vi "PID_controller_21.vi"() -> ()   [LabVIEW 2011]
uses:
  <vilib>/Analysis/NI_AALPro.lvlib
panel:
  in  "|angle backlash|":dbl
  out "prev dAngle":dbl
  out "dAngle":dbl
  out "XY Graph 2":cluster{"Value":dbl[], "Value":dbl[]}(graph)
  out "Angle array":dbl[](array[numeric])
  in  "Move to ref angle first":bool=TRUE
  in  "time to wait (s)":dbl=2.0
  in  "angle backlash (deg)":dbl=5.0 format="%.1f"
  out "Polynomial Coefficients":dbl[](array[numeric])=[-1.4185856873488687, 0.3207828308209371, 0.13144453708617976]
  out "Best Polynomial Fit":dbl[](array[numeric])=[-1.4185856873488687, -1.6139263817489564, -1.4535753275096295, -0.934721257482187, -0.06084472416107456, 1.168009538292087, 2.7539547788012695, 4.6979090060566655, 6.9965349595828625, 9.65378216839643, 12.656869913925354, 16.032582856357365, 19.766321537116767, 23.839791139200322, 28.29201256813708, 33.090057519195085, 38.231169600301214, 43.741895001434145, 49.604230522561835, 55.817258155180305, 63.621549699110574, 70.69684374251437, 78.07805746158404, 85.78401348130417, 93.89514333055536, 102.37353612475415, 111.1585051750553, 120.33168859799997, 129.86351160527155, 139.71949074374146, 149.9584374415381, 160.56464392932688, 171.50086747103902, 182.82343196442633, 194.50463604214053, 206.47125485701025, 218.94296295023602, 231.70008578092185, 244.74755627283324, 258.3136303817438]
  out "tFit_array":dbl[](array[numeric])=[-2.0, 0.0]
  out "PFit_array":dbl[](array[numeric])=[73.96843433835814, 74.61000000000001]
  out "error array":dbl[](array[numeric])=[-1.3899999999999864, -1.7800000000000011, -1.3500000000000085, -0.6200000000000045, 0.5699999999999932, 1.6099999999999994, 1.1999999999999886, 0.3199999999999932, -0.13000000000000966, -1.3700000000000045, -1.9499999999999886, -1.7399999999999949, -1.1200000000000045, -0.11999999999999034, 1.759999999999991, 2.3500000000000085, 2.1700000000000017, 1.4099999999999966, 0.4299999999999926, -0.6500000000000057, 54.959999999999994, 55.099999999999994, 55.66000000000001, 56.55000000000001, 57.02000000000001, 58.03, 58.129999999999995, 57.11999999999999, 56.599999999999994, 55.47, 54.80000000000001, 54.84, 55.129999999999995, 55.58, 57.16000000000001, 58.11, 58.09, 57.510000000000005, 56.74000000000001, 55.709999999999994]
  out "dt array":dbl[](array[numeric])=[0.0, -1.1669999999867287, -2.3260000000009313, -3.4940000000060536, -4.657999999995809, -5.820999999996275, -6.98499999998603, -8.14999999999418, -9.314000000013039, -10.478999999992084, -11.64000000001397, -12.807000000000698, -13.973999999987427, -15.135999999998603, -16.304000000003725, -17.469000000011874, -18.630999999993946, -19.796000000002095, -20.95999999999185, -22.122999999992317, -23.497999999992317, -24.67499999998836, -25.84299999999348, -27.005999999993946, -28.176000000006752, -29.347000000008848, -30.510999999998603, -31.679000000003725, -32.84700000000885, -34.0109999999986, -35.178000000014435, -36.345999999990454, -37.5109999999986, -38.679000000003725, -39.84700000000885, -41.00800000000163, -42.18299999998999, -43.35099999999511, -44.513000000006286, -45.68900000001304]
  out "Pset array":dbl[](array[numeric])=[76.0, 76.0, 76.0, 76.0, 76.0, 76.0, 76.0, 76.0, 76.0, 76.0, 76.0, 76.0, 76.0, 76.0, 76.0, 76.0, 76.0, 76.0, 76.0, 76.0, 20.0, 20.0, 20.0, 20.0, 20.0, 20.0, 20.0, 20.0, 20.0, 20.0, 20.0, 20.0, 20.0, 20.0, 20.0, 20.0, 20.0, 20.0, 20.0, 20.0]
  out "t array":dbl[](array[numeric])=[161845.394, 161844.227, 161843.068, 161841.9, 161840.736, 161839.573, 161838.409, 161837.244, 161836.08, 161834.915, 161833.754, 161832.587, 161831.42, 161830.258, 161829.09, 161827.925, 161826.763, 161825.598, 161824.434, 161823.271, 161821.896, 161820.719, 161819.551, 161818.388, 161817.218, 161816.047, 161814.883, 161813.715, 161812.547, 161811.383, 161810.216, 161809.048, 161807.883, 161806.715, 161805.547, 161804.386, 161803.211, 161802.043, 161800.881, 161799.705]
  out "P array":dbl[](array[numeric])=[74.61000000000001, 74.22, 74.64999999999999, 75.38, 76.57, 77.61, 77.19999999999999, 76.32, 75.86999999999999, 74.63, 74.05000000000001, 74.26, 74.88, 75.88000000000001, 77.75999999999999, 78.35000000000001, 78.17, 77.41, 76.42999999999999, 75.35, 74.96, 75.1, 75.66000000000001, 76.55000000000001, 77.02000000000001, 78.03, 78.13, 77.11999999999999, 76.6, 75.47, 74.80000000000001, 74.84, 75.13, 75.58, 77.16000000000001, 78.11, 78.09, 77.51, 76.74000000000001, 75.71]
  in  "Local":bool
  in  "Hold":bool
  out "tune_Method":u16(ring)=1 items=["Setpoint", "Angle"]
  in  "Method":u16(ring)=1 items=["Setpoint", "Angle"]
  in  "Setpoint":u16(ring) items=["A", "B", "C", "D"]
  out "tuning":bool
  in  "Tune":bool
  out "Tune Set Point (torr)":dbl=76.0 format="%.2f"
  in  "stop":bool
  out "err_avg":dbl=-1.1485673305631505
  out "Setpoint":string="A"
  in  "Ks":dbl
  out "dt(s)":dbl=1.1669999999867287
  out "windup error":dbl
  out "tPrev":dbl=161845.394
  out "target value":dbl=8.607079070006002
  out "error":dbl=-1.3899999999999864
  out "tStart(s)":dbl=161845.394
  out "weight array":dbl[](array[numeric])=[1.0, 0.3112994401423479, 0.09768570948263659, 0.03037911236430853, 0.009485414272106564, 0.0029646390229553033, 0.0009256632966347818, 0.00028873535962988374, 9.01532101455707e-05, 2.8120829299984297e-05, 8.806680295207305e-06, 2.741514645410681e-06, 8.534319742583924e-07, 2.6700458671159456e-07, 8.303530152421186e-08, 2.5900592293904588e-08, 8.103255033572197e-09, 2.5275888811806865e-09, 7.892010589399871e-10, 2.4666252724157755e-10, 6.236605368793774e-11, 1.9221339918994332e-11, 5.977611753902341e-12, 1.8682854076081917e-12, 5.79854027362869e-13, 1.7978764328562998e-13, 5.613594818436806e-14, 1.74576228867237e-14, 5.429116398891195e-15, 1.6951587510987664e-15, 5.277019701540894e-16, 1.6410913665416056e-16, 5.1189358768628024e-17, 1.5919291471855112e-17, 4.95071333304516e-18, 1.5504290109481995e-18, 4.788019052453027e-19, 1.4890178877471836e-19, 4.6585389077974155e-20, 1.437207306183795e-20]
  in  "# of points to watch":i32=60
  in  "tSmooth(s)":dbl=1.0
  out "IO error":errorcluster
  out "first":bool
  out "XY Graph":cluster{"Value":dbl[], "Value":dbl[]}[](graph)=[{"Value"=[0.0, -1.1669999999867287, -2.3260000000009313, -3.4940000000060536, -4.657999999995809, -5.820999999996275, -6.98499999998603, -8.14999999999418, -9.314000000013039, -10.478999999992084, -11.64000000001397, -12.807000000000698, -13.973999999987427, -15.135999999998603, -16.304000000003725, -17.469000000011874, -18.630999999993946, -19.796000000002095, -20.95999999999185, -22.122999999992317, -23.497999999992317, -24.67499999998836, -25.84299999999348, -27.005999999993946, -28.176000000006752, -29.347000000008848, -30.510999999998603, -31.679000000003725, -32.84700000000885, -34.0109999999986, -35.178000000014435, -36.345999999990454, -37.5109999999986, -38.679000000003725, -39.84700000000885, -41.00800000000163, -42.18299999998999, -43.35099999999511, -44.513000000006286, -45.68900000001304], "Value"=[74.61000000000001, 74.22, 74.64999999999999, 75.38, 76.57, 77.61, 77.19999999999999, 76.32, 75.86999999999999, 74.63, 74.05000000000001, 74.26, 74.88, 75.88000000000001, 77.75999999999999, 78.35000000000001, 78.17, 77.41, 76.42999999999999, 75.35, 74.96, 75.1, 75.66000000000001, 76.55000000000001, 77.02000000000001, 78.03, 78.13, 77.11999999999999, 76.6, 75.47, 74.80000000000001, 74.84, 75.13, 75.58, 77.16000000000001, 78.11, 78.09, 77.51, 76.74000000000001, 75.71]}, {"Value"=[-2.0, 0.0], "Value"=[73.96843433835814, 74.61000000000001]}, {"Value"=[0.0, -1.1669999999867287, -2.3260000000009313, -3.4940000000060536, -4.657999999995809, -5.820999999996275, -6.98499999998603, -8.14999999999418, -9.314000000013039, -10.478999999992084, -11.64000000001397, -12.807000000000698, -13.973999999987427, -15.135999999998603, -16.304000000003725, -17.469000000011874, -18.630999999993946, -19.796000000002095, -20.95999999999185, -22.122999999992317, -23.497999999992317, -24.67499999998836, -25.84299999999348, -27.005999999993946, -28.176000000006752, -29.347000000008848, -30.510999999998603, -31.679000000003725, -32.84700000000885, -34.0109999999986, -35.178000000014435, -36.345999999990454, -37.5109999999986, -38.679000000003725, -39.84700000000885, -41.00800000000163, -42.18299999998999, -43.35099999999511, -44.513000000006286, -45.68900000001304], "Value"=[76.0, 76.0, 76.0, 76.0, 76.0, 76.0, 76.0, 76.0, 76.0, 76.0, 76.0, 76.0, 76.0, 76.0, 76.0, 76.0, 76.0, 76.0, 76.0, 76.0, 20.0, 20.0, 20.0, 20.0, 20.0, 20.0, 20.0, 20.0, 20.0, 20.0, 20.0, 20.0, 20.0, 20.0, 20.0, 20.0, 20.0, 20.0, 20.0, 20.0]}]
  out "current value":dbl=8.607079070006002
  in  "Period (s)":dbl=0.5
  out "dValue":dbl=2.1714937580001004
  out "derivative":dbl=0.3207828308209371
  out "integral":dbl=21701.037580001004
  in  "Angle (deg)":dbl=20.3 format="%.1f"
  in  "Kd":dbl
  in  "Ki":dbl=0.0001
  in  "Kp":dbl=0.001
  out "P (torr)":dbl=74.61000000000001 format="%.2f"
  in  "Set Point (torr)":dbl=76.0 format="%.2f"
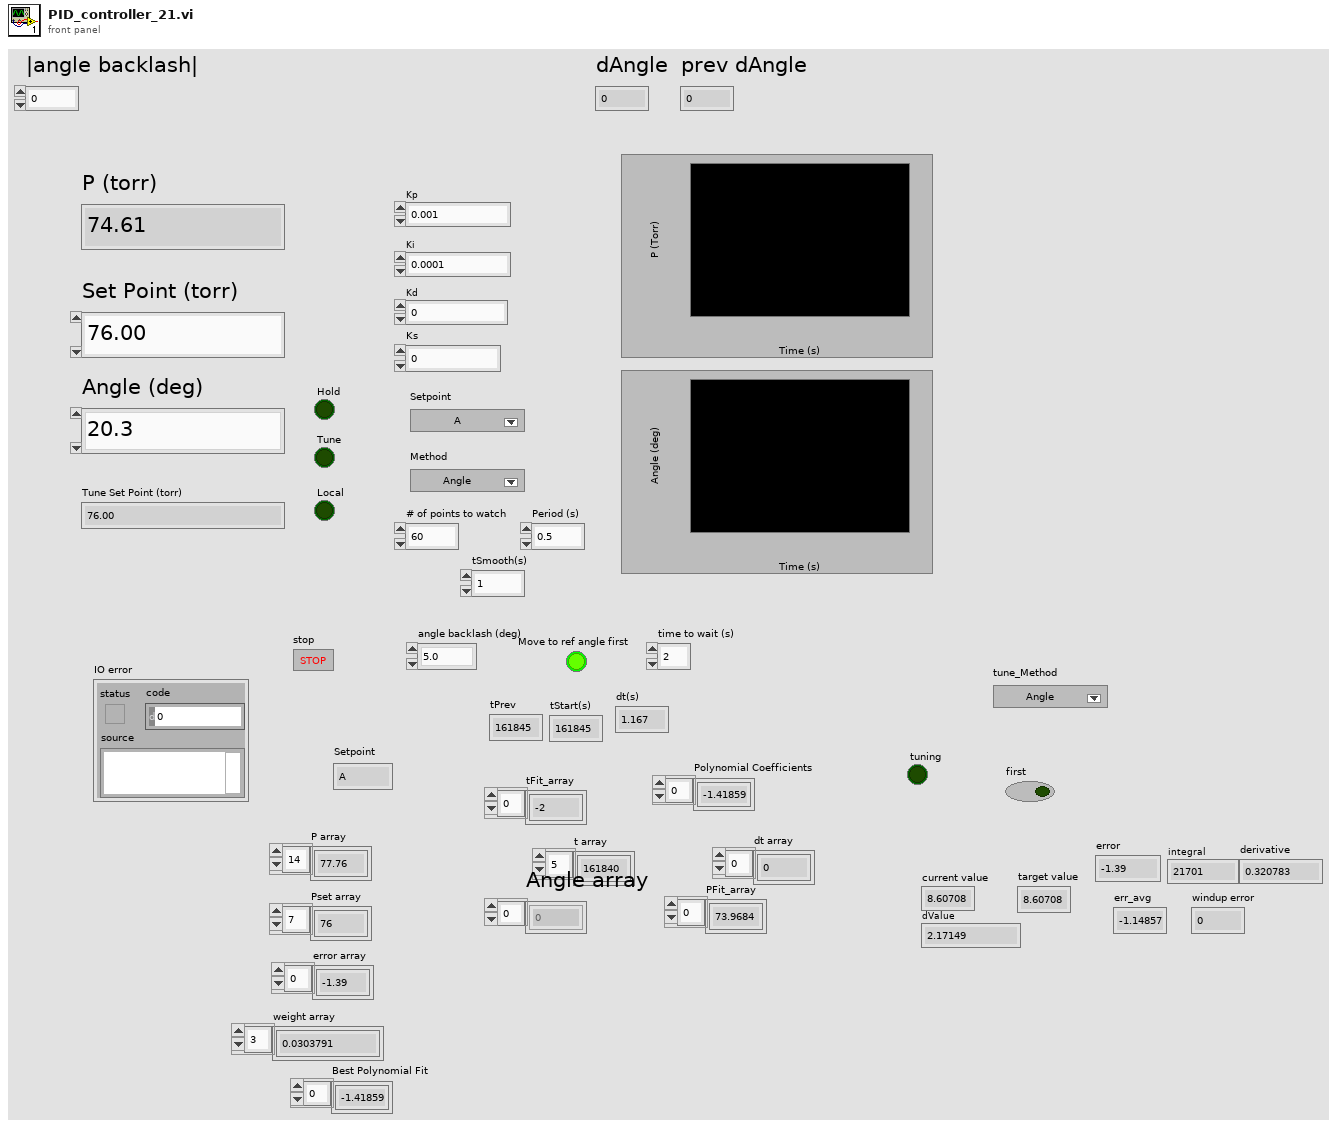
[diagram p1: front panel]
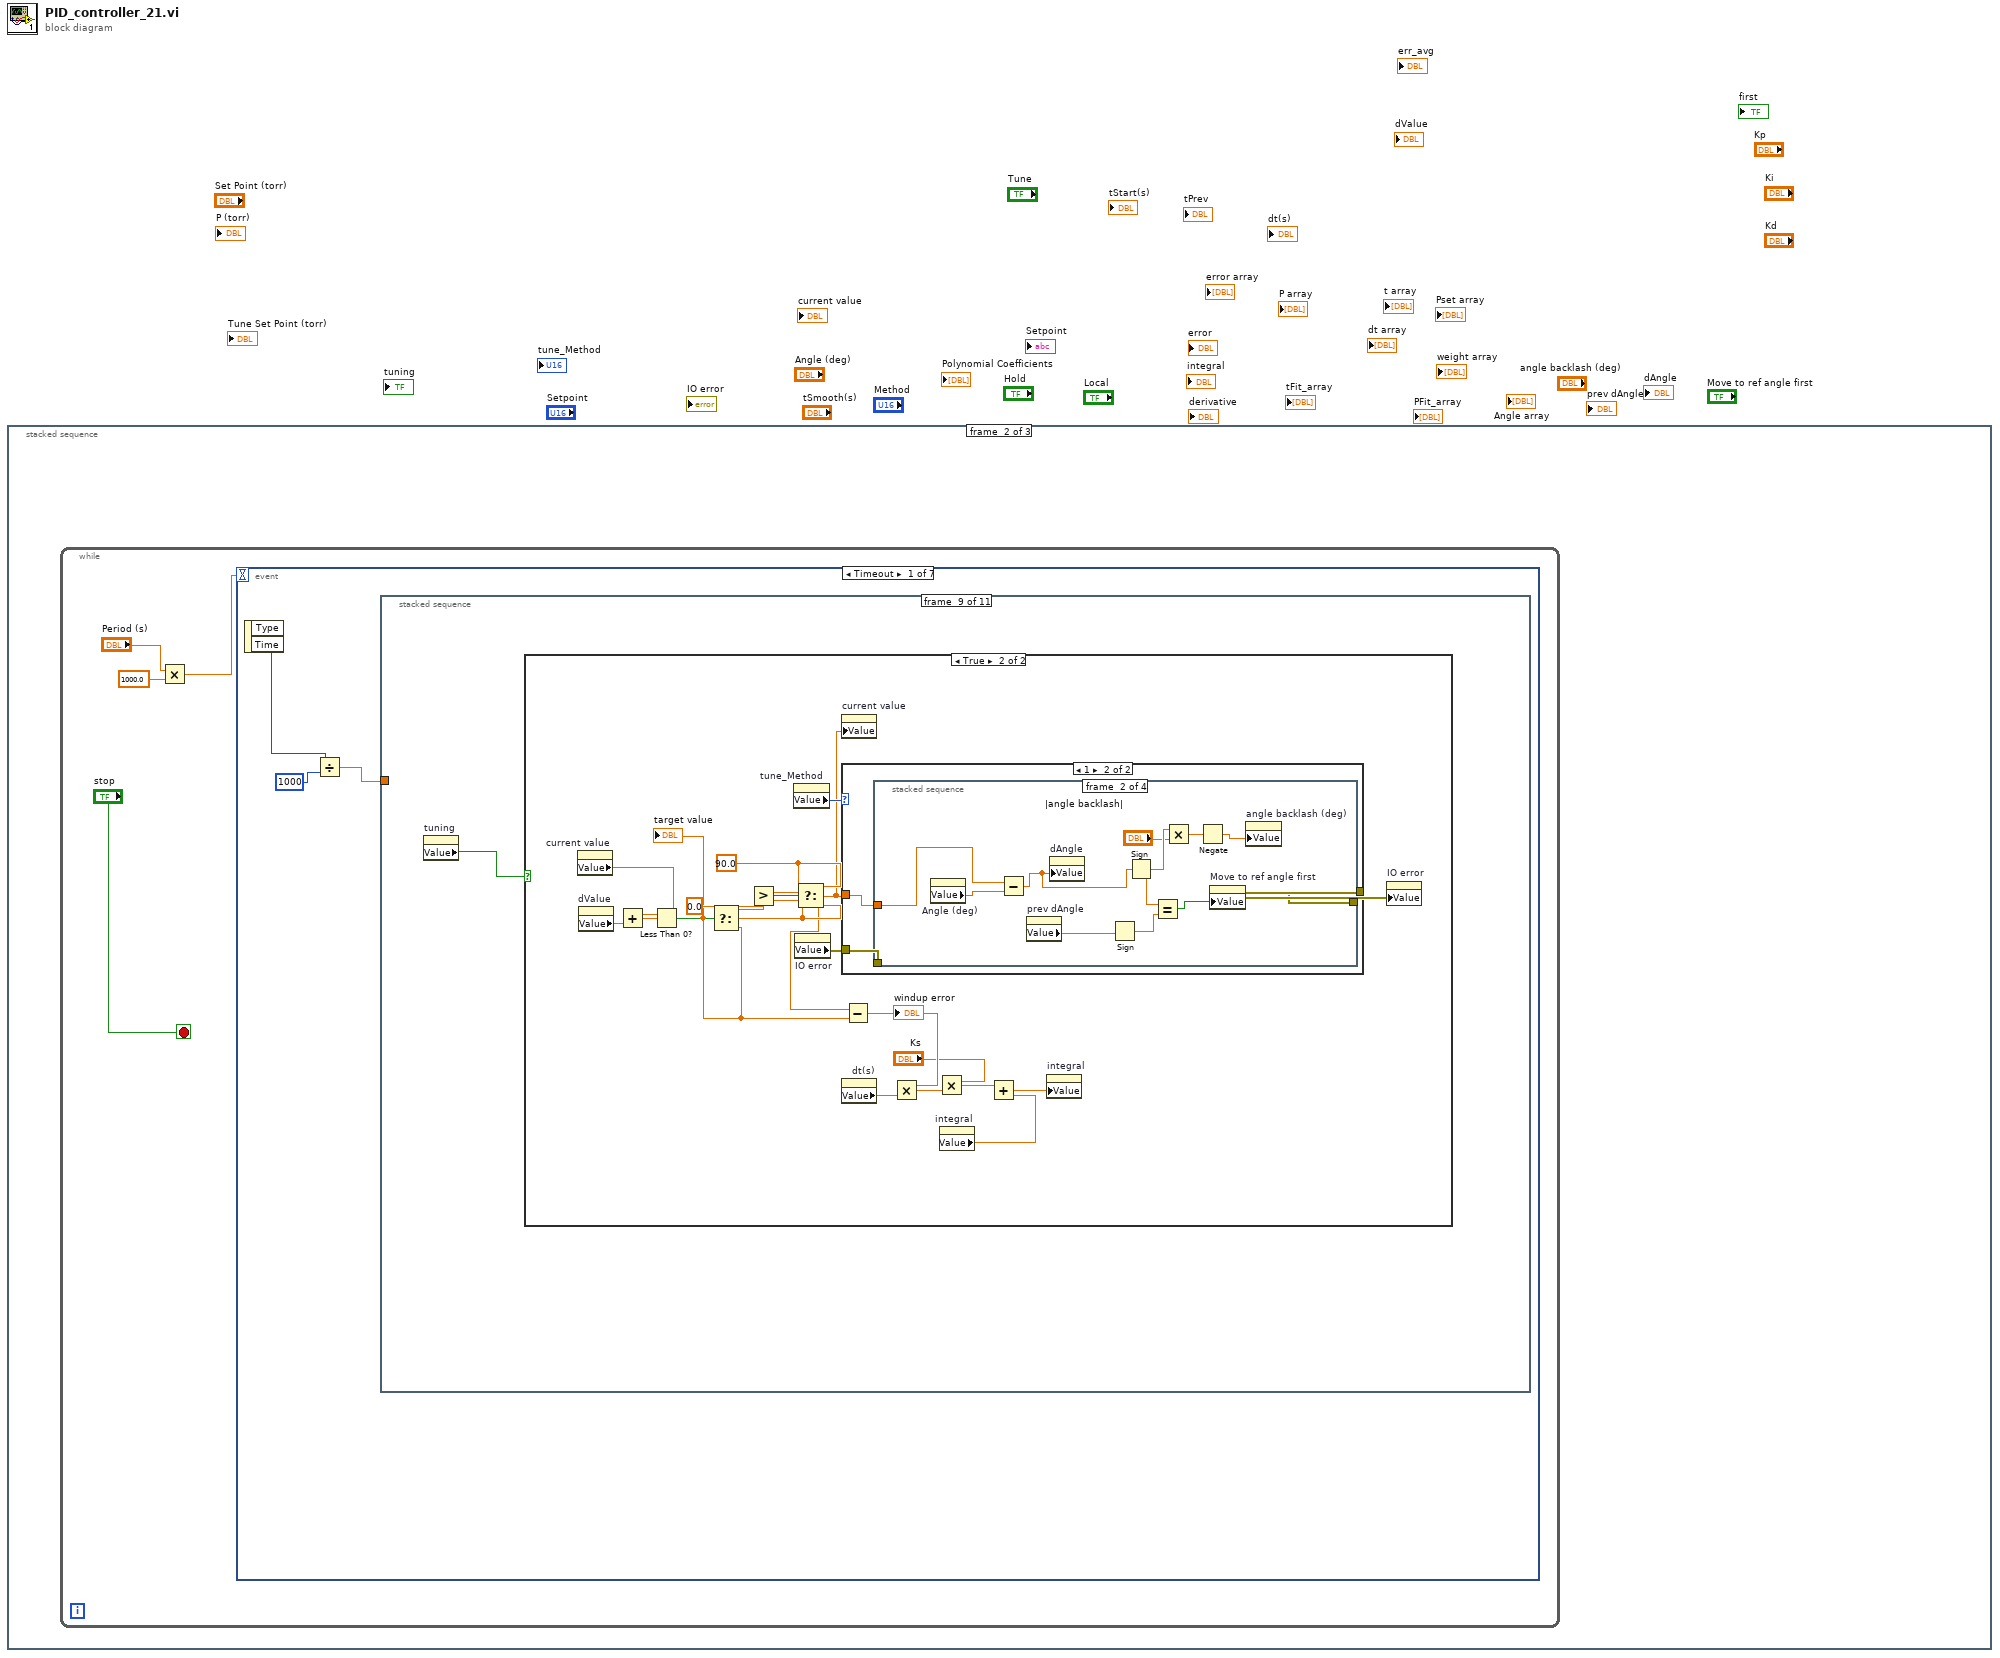
[diagram p0: block diagram]
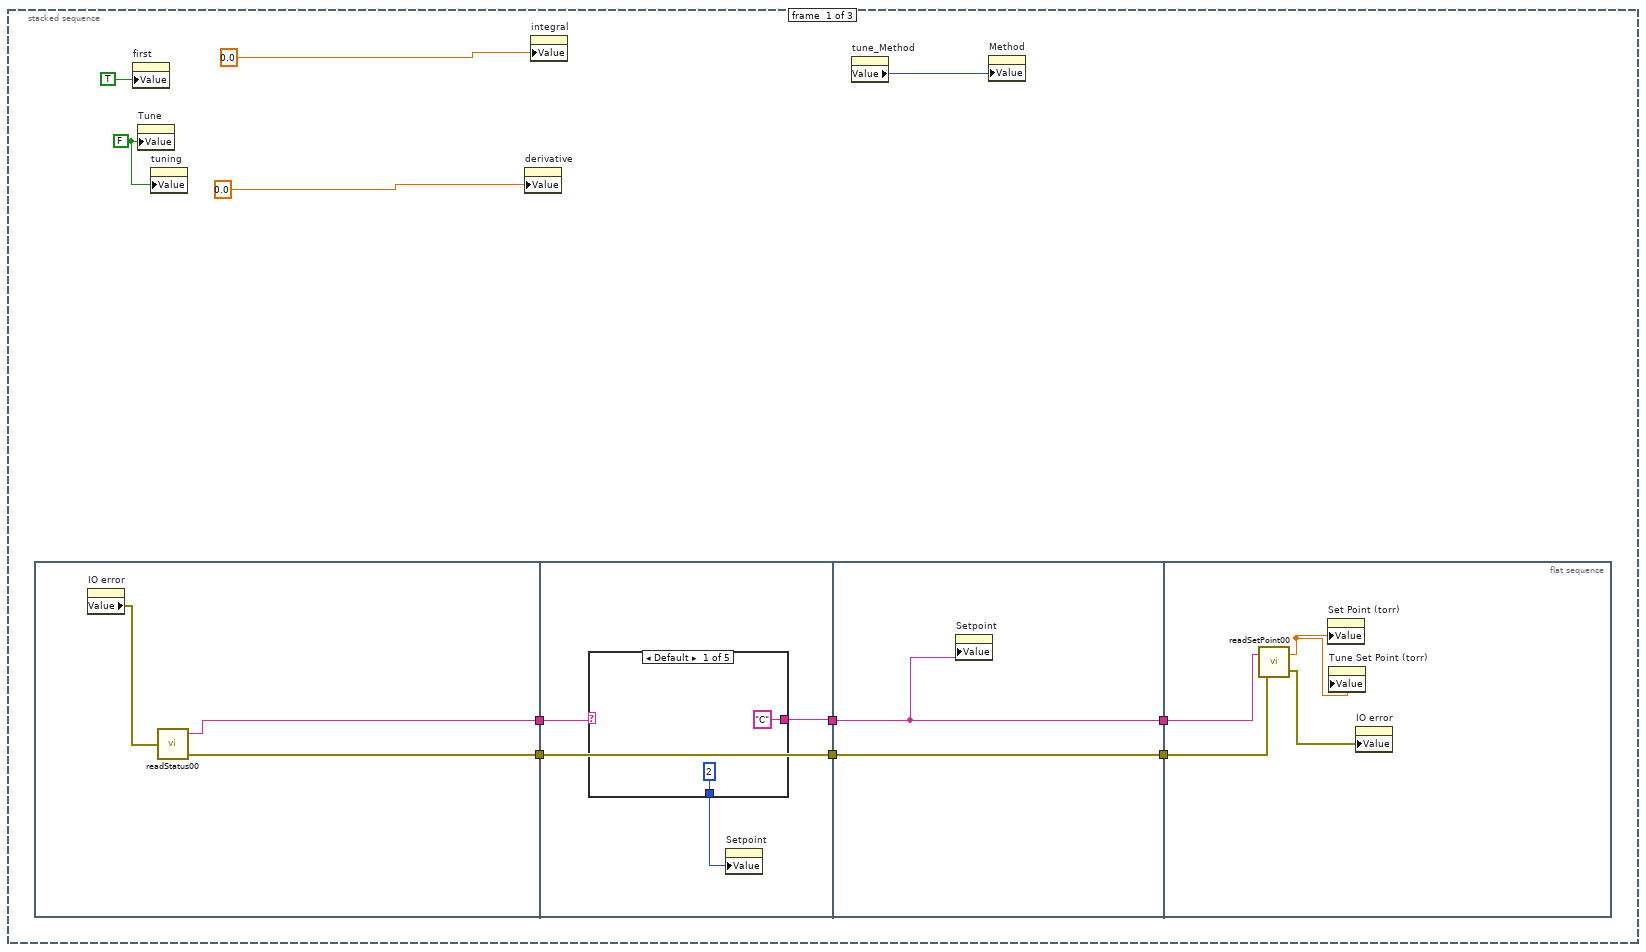
[diagram p2: hidden frame]
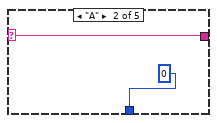
[diagram p3: hidden frame]
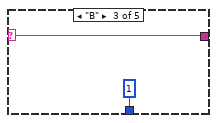
[diagram p4: hidden frame]
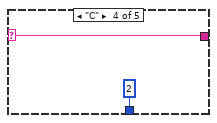
[diagram p5: hidden frame]
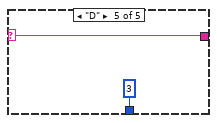
[diagram p6: hidden frame]
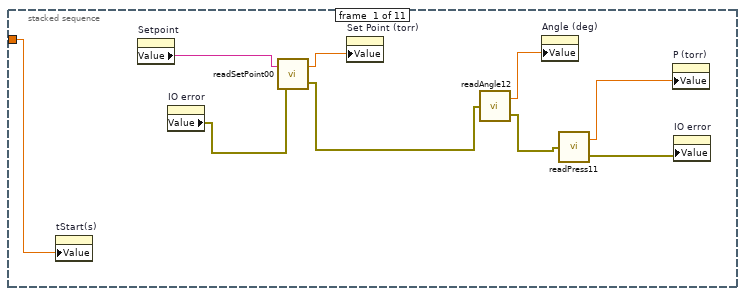
[diagram p7: hidden frame]
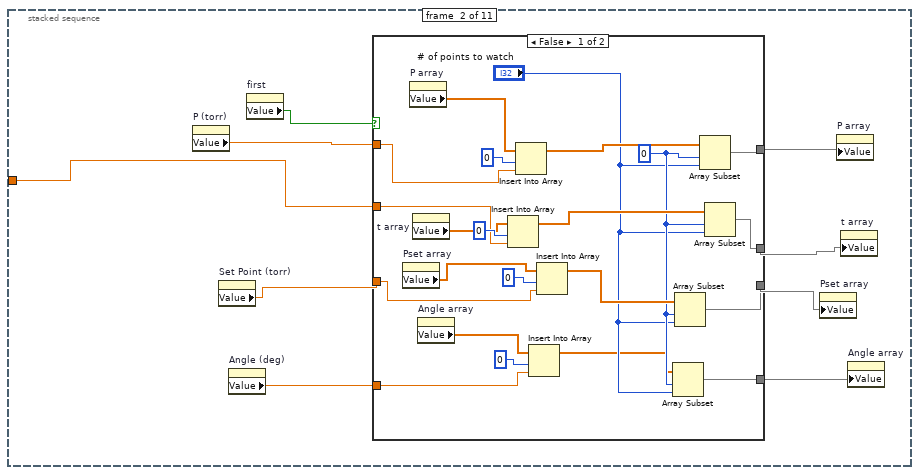
[diagram p8: hidden frame]
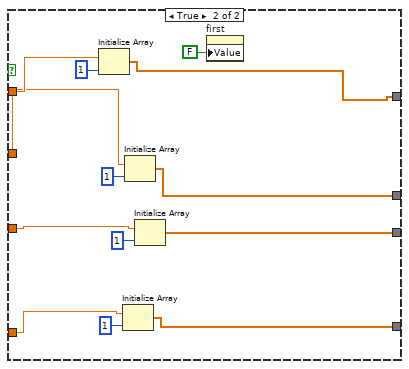
[diagram p9: hidden frame]
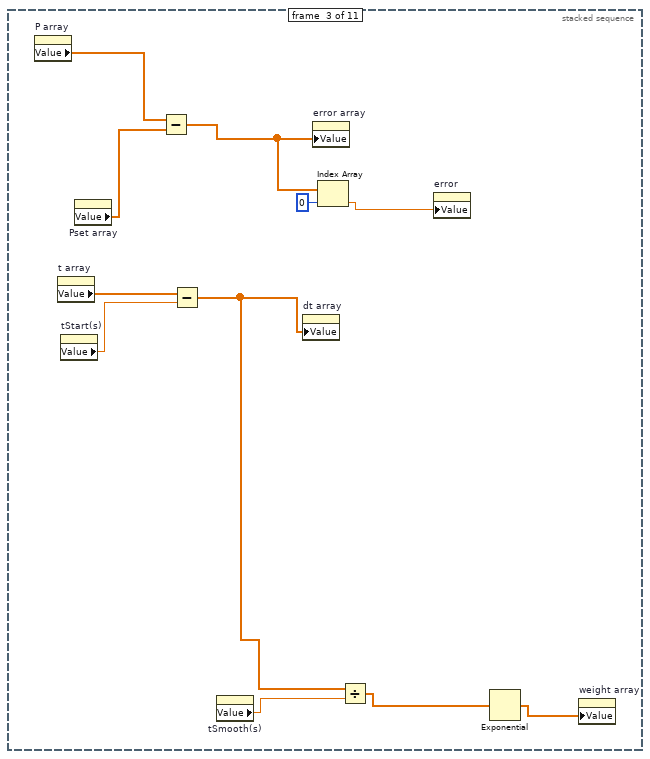
[diagram p10: hidden frame]
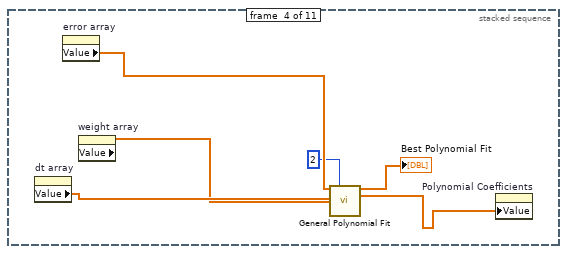
[diagram p11: hidden frame]
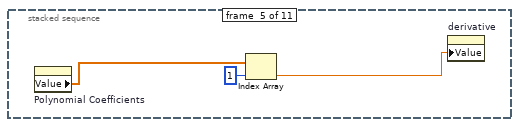
[diagram p12: hidden frame]
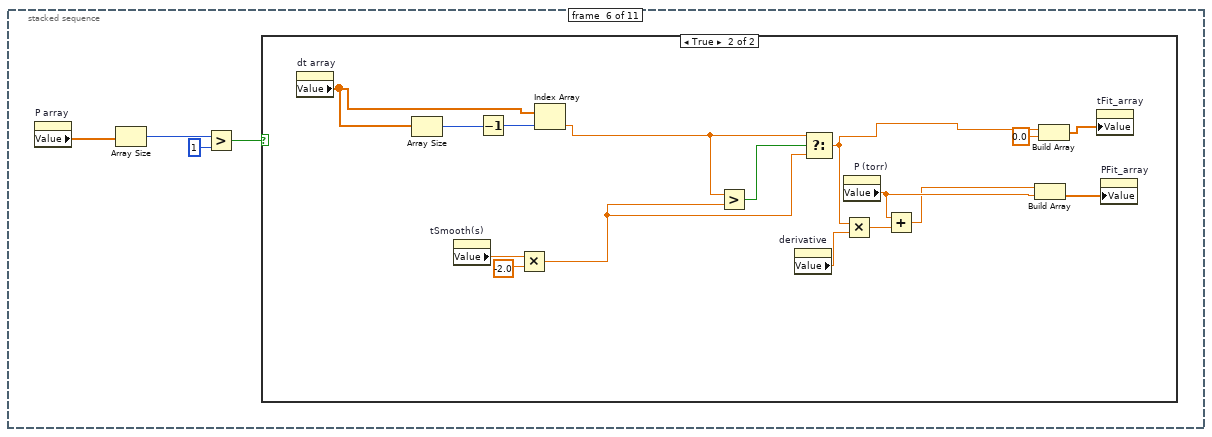
[diagram p13: hidden frame]
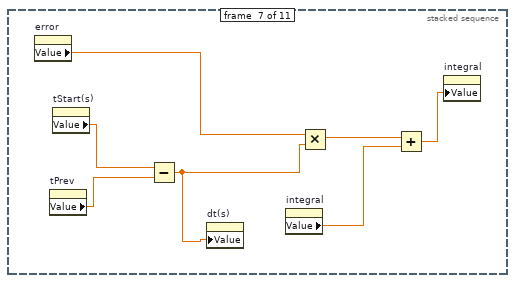
[diagram p15: hidden frame]
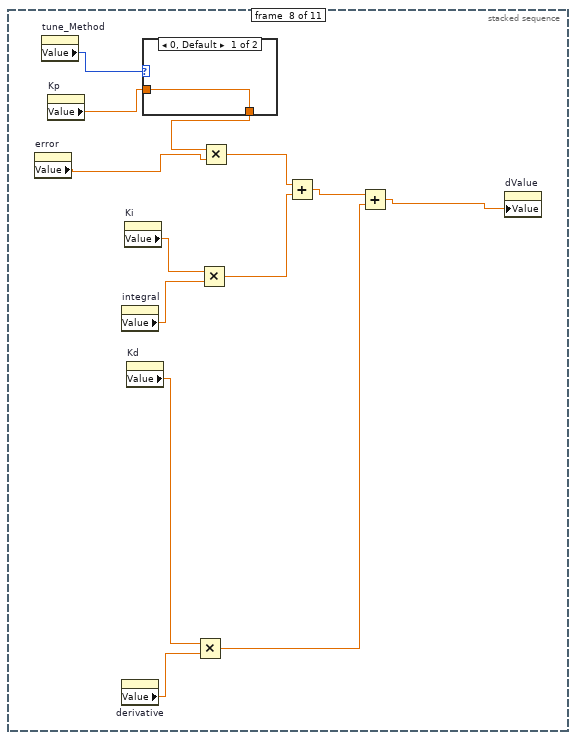
[diagram p16: hidden frame]
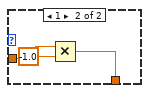
[diagram p17: hidden frame]
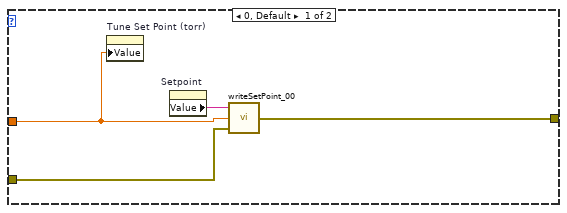
[diagram p19: hidden frame]
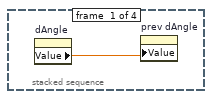
[diagram p20: hidden frame]
diagram:
  n1 = stacked-sequence {
    frame #0 {
      w8 = FALSE ("Tune")
      n2 = flat-sequence {
        tunnel: [w13] -> w7
        tunnel: [w12] -> w6
        tunnel: w7 -> [w17]
        tunnel: [w16] -> w5
        tunnel: w6 -> [w18]
        tunnel: [w18] -> w3
        tunnel: w5 -> [w29]
        tunnel: [w29] -> w4
        tunnel: w3 -> [w30]
        tunnel: [w30] -> w2
        tunnel: w4 -> [w34]
        tunnel: w2 -> [w33]
        frame #0 {
          n3 = property on="IO error" class="Clust (strict)"() -> ("Value"=w14:errorcluster)  [unwired: 2 in, 2 out]
          n4 = call "readStatus00.vi"("error in"=w14) -> ("Setpoint"=w13:string, "error out"=w12:errorcluster)  [unwired: 1 out]
        }
        frame #1 {
          n5 = case shown="Default" w17 {
            selector: w17 -> [_ w22 w23 w25 w27]
            tunnel: ["C" w22 w23 w25 w27] -> w16
            tunnel: [u16 2 ("Ring") u16 0 ("Ring") u16 1 ("Ring") u16 2 ("Ring") u16 3 ("Ring")] -> w15
            frame Default {
            }
            frame "A" {
            }
            frame "B" {
            }
            frame "C" {
            }
            frame "D" {
            }
          }
          n6 = property on="Setpoint" class="Ring (strict)"("Value"=w15) -> ()  [unwired: 2 in, 2 out]
        }
        frame #2 {
          n7 = property on="Setpoint" class="Str"("Value"=w29) -> ()  [unwired: 2 in, 2 out]
        }
        frame #3 {
          n8 = call "readSetPoint00.vi"("error in"=w33, "Setpoint"=w34) -> ("error out"=w32:errorcluster, "P"=w31:dbl)
          n9 = property on="Set Point (torr)" class="DigNum (strict)"("Value"=w31) -> ()  [unwired: 2 in, 2 out]
          n10 = property on="Tune Set Point (torr)" class="DigNum (strict)"("Value"=w31) -> ()  [unwired: 2 in, 2 out]
          n11 = property on="IO error" class="Clust (strict)"("Value"=w32) -> ()  [unwired: 2 in, 2 out]
        }
      }
      n12 = property on="first" class="Bool (strict)"("Value"=TRUE ("first")) -> ()  [unwired: 2 in, 2 out]
      n13 = property on="Tune" class="Bool (strict)"("Value"=w8) -> ()  [unwired: 2 in, 2 out]
      n14 = property on="tuning" class="Bool (strict)"("Value"=w8) -> ()  [unwired: 2 in, 2 out]
      n15 = property on="derivative" class="DigNum (strict)"("Value"=0.0 ("derivative")) -> ()  [unwired: 2 in, 2 out]
      n16 = property on="integral" class="DigNum (strict)"("Value"=0.0 ("integral")) -> ()  [unwired: 2 in, 2 out]
      n17 = property on="tune_Method" class="Ring (strict)"() -> ("Value"=w1:u16)  [unwired: 2 in, 2 out]
      n18 = property on="Method" class="Ring (strict)"("Value"=w1) -> ()  [unwired: 2 in, 2 out]
    }
    frame #1 {
      n19 = while {
        stop <- "stop" stop-if-true
        n20 = Multiply(x="Period (s)", y=1000.0) -> (x*y=w36:dbl)
        n21 = event shown="[0] Timeout" {
          selector: _ -> [_ _ _ _ _ _ _]
          dyn-events: _ -> [_ _ _ _ _ _ _]
          timeout: w36 -> [_ _ _ _ _ _ _]
          event Timeout {
            n22 = event-data() -> ("Time"=w41:u32)  [unwired: 1 in, 1 out]
            n23 = Divide(x=w41, y=u32 1000) -> (x/y=w39:dbl)
            n24 = stacked-sequence {
              tunnel: w39 -> [w45 w59 _ _ _ _ _ _ _ _ _]
              frame #0 {
                n25 = property on="tStart(s)" class="DigNum (strict)"("Value"=w45) -> ()  [unwired: 2 in, 2 out]
                n26 = property on="Setpoint" class="Str"() -> ("Value"=w48:string)  [unwired: 2 in, 2 out]
                n27 = property on="IO error" class="Clust (strict)"() -> ("Value"=w49:errorcluster)  [unwired: 2 in, 2 out]
                n28 = call "readSetPoint00.vi"("error in"=w49, "Setpoint"=w48) -> ("error out"=w47:errorcluster, "P"=w50:dbl)
                n29 = property on="Set Point (torr)" class="DigNum (strict)"("Value"=w50) -> ()  [unwired: 2 in, 2 out]
                n30 = call "readAngle12.vi"("error in"=w47) -> ("angle"=w46:dbl, "error out"=w44:errorcluster)
                n31 = property on="Angle (deg)" class="DigNum (strict)"("Value"=w46) -> ()  [unwired: 2 in, 2 out]
                n32 = call "readPress11.vi"("error in"=w44) -> ("P"=w42:dbl, "error out"=w43:errorcluster)
                n33 = property on="P (torr)" class="DigNum (strict)"("Value"=w42) -> ()  [unwired: 2 in, 2 out]
                n34 = property on="IO error" class="Clust (strict)"("Value"=w43) -> ()  [unwired: 2 in, 2 out]
              }
              frame #1 {
                n35 = property on="P (torr)" class="DigNum (strict)"() -> ("Value"=w57:dbl)  [unwired: 2 in, 2 out]
                n36 = property on="Set Point (torr)" class="DigNum (strict)"() -> ("Value"=w54:dbl)  [unwired: 2 in, 2 out]
                n37 = property on="Angle (deg)" class="DigNum (strict)"() -> ("Value"=w52:dbl)  [unwired: 2 in, 2 out]
                n38 = property on="first" class="Bool (strict)"() -> ("Value"=w58:bool)  [unwired: 2 in, 2 out]
                n39 = case shown="False" w58 {
                  tunnel: w57 -> [w80 w93]
                  tunnel: [w71 w91] -> w56
                  tunnel: w59 -> [w77 w89]
                  tunnel: [w69 w88] -> w55
                  tunnel: w54 -> [w73 w86]
                  tunnel: [w67 w85] -> w53
                  tunnel: w52 -> [w66 w83]
                  tunnel: [w61 w82] -> w51
                  frame False {
                    w64 = 0 ("index")
                    n40 = property on="Pset array" class="Arr (strict)"() -> ("Value"=w74:dbl[])  [unwired: 2 in, 2 out]
                    n41 = property on="P array" class="Arr (strict)"() -> ("Value"=w79:dbl[])  [unwired: 2 in, 2 out]
                    n42 = property on="t array" class="Arr (strict)"() -> ("Value"=w76:dbl[])  [unwired: 2 in, 2 out]
                    n43 = property on="Angle array" class="Arr (strict)"() -> ("Value"=w65:dbl[])  [unwired: 2 in, 2 out]
                    n44 = Insert Into Array(array=w76, index=0, new element=w77) -> (w70:dbl[])
                    n45 = Insert Into Array(array=w79, index=0, new element=w80) -> (w72:dbl[])
                    n46 = Insert Into Array(array=w65, index=0, new element=w66) -> (w62:dbl[])
                    n47 = Insert Into Array(array=w74, index=0, new element=w73) -> (w68:dbl[])
                    n48 = Array Subset(array=w62, index=w64, length="# of points to watch") -> (w61:dbl[])
                    n49 = Array Subset(array=w68, index=w64, length="# of points to watch") -> (w67:dbl[])
                    n50 = Array Subset(array=w72, index=w64, length="# of points to watch") -> (w71:dbl[])
                    n51 = Array Subset(array=w70, index=w64, length="# of points to watch") -> (w69:dbl[])
                  }
                  frame True {
                    n52 = Initialize Array(w93, 1 ("dimension size")) -> (w91:dbl[])
                    n53 = Initialize Array(w83, 1 ("dimension size")) -> (w82:dbl[])
                    n54 = Initialize Array(w89, 1 ("dimension size")) -> (w88:dbl[])
                    n55 = Initialize Array(w86, 1 ("dimension size")) -> (w85:dbl[])
                    n56 = property on="first" class="Bool (strict)"("Value"=FALSE ("first")) -> ()  [unwired: 2 in, 2 out]
                  }
                }
                n57 = property on="Pset array" class="Arr (strict)"("Value"=w53) -> ()  [unwired: 2 in, 2 out]
                n58 = property on="P array" class="Arr (strict)"("Value"=w56) -> ()  [unwired: 2 in, 2 out]
                n59 = property on="t array" class="Arr (strict)"("Value"=w55) -> ()  [unwired: 2 in, 2 out]
                n60 = property on="Angle array" class="Arr (strict)"("Value"=w51) -> ()  [unwired: 2 in, 2 out]
              }
              frame #2 {
                n61 = property on="P array" class="Arr (strict)"() -> ("Value"=w99:dbl[])  [unwired: 2 in, 2 out]
                n62 = property on="t array" class="Arr (strict)"() -> ("Value"=w105:dbl[])  [unwired: 2 in, 2 out]
                n63 = property on="tStart(s)" class="DigNum (strict)"() -> ("Value"=w104:dbl)  [unwired: 2 in, 2 out]
                n64 = property on="Pset array" class="Arr (strict)"() -> ("Value"=w98:dbl[])  [unwired: 2 in, 2 out]
                n65 = Subtract(x=w99, y=w98) -> (x-y=w97:dbl[])
                n66 = Subtract(x=w105, y=w104) -> (x-y=w101:dbl[])
                n67 = property on="tSmooth(s)" class="DigNum (strict)"() -> ("Value"=w103:dbl)  [unwired: 2 in, 2 out]
                n68 = property on="dt array" class="Arr (strict)"("Value"=w101) -> ()  [unwired: 2 in, 2 out]
                n69 = property on="error array" class="Arr (strict)"("Value"=w97) -> ()  [unwired: 2 in, 2 out]
                n70 = Index Array(array=w97, index=0) -> (element=w95:dbl)
                n71 = Divide(x=w101, y=w103) -> (x/y=w102:dbl[])
                n72 = property on="error" class="DigNum (strict)"("Value"=w95) -> ()  [unwired: 2 in, 2 out]
                n73 = Exponential(1:w102) -> (0:w100:dbl[])
                n74 = property on="weight array" class="Arr (strict)"("Value"=w100) -> ()  [unwired: 2 in, 2 out]
              }
              frame #3 {
                n75 = property on="dt array" class="Arr (strict)"() -> ("Value"=w110:dbl[])  [unwired: 2 in, 2 out]
                n76 = property on="error array" class="Arr (strict)"() -> ("Value"=w111:dbl[])  [unwired: 2 in, 2 out]
                n77 = property on="weight array" class="Arr (strict)"() -> ("Value"=w109:dbl[])  [unwired: 2 in, 2 out]
                n78 = call <vilib>:"General Polynomial Fit.vi"("Y"=w111, "polynomial order"=2, "X"=w110, "Weight"=w109) -> ("Best Polynomial Fit"=→"Best Polynomial Fit":dbl[], "Polynomial Coefficients"=w106:dbl[])  [unwired: 8 in, 2 out]
                n79 = property on="Polynomial Coefficients" class="Arr (strict)"("Value"=w106) -> ()  [unwired: 2 in, 2 out]
              }
              frame #4 {
                n80 = property on="Polynomial Coefficients" class="Arr (strict)"() -> ("Value"=w114:dbl[])  [unwired: 2 in, 2 out]
                n81 = Index Array(array=w114, index=1) -> (element=w112:dbl)
                n82 = property on="derivative" class="DigNum (strict)"("Value"=w112) -> ()  [unwired: 2 in, 2 out]
              }
              frame #5 {
                n83 = property on="P array" class="Arr (strict)"() -> ("Value"=w115:dbl[])  [unwired: 2 in, 2 out]
                n84 = Array Size(array=w115) -> (size(s)=w116:i32)
                n85 = Greater?(x=w116, y=1) -> (0:w118:bool)
                n86 = case shown="True" w118 {
                  frame False {
                  }
                  frame True {
                    n87 = property on="dt array" class="Arr (strict)"() -> ("Value"=w126:dbl[])  [unwired: 2 in, 2 out]
                    n88 = Array Size(array=w126) -> (size(s)=w134:i32)
                    n89 = property on="tSmooth(s)" class="DigNum (strict)"() -> ("Value"=w128:dbl)  [unwired: 2 in, 2 out]
                    n90 = Decrement(x=w134) -> (x-1=w133:i32)
                    n91 = Multiply(x=w128, y=-2.0) -> (x*y=w119:dbl)
                    n92 = Index Array(array=w126, index=w133) -> (element=w127:dbl)
                    n93 = Greater?(x=w127, y=w119) -> (0:w130:bool)
                    n94 = property on="derivative" class="DigNum (strict)"() -> ("Value"=w132:dbl)  [unwired: 2 in, 2 out]
                    n95 = Select(t=w127, s=w130, f=w119) -> (s? t:f=w123:dbl)
                    n96 = property on="P (torr)" class="DigNum (strict)"() -> ("Value"=w125:dbl)  [unwired: 2 in, 2 out]
                    n97 = Multiply(x=w123, y=w132) -> (x*y=w131:dbl)
                    n98 = Add(x=w125, y=w131) -> (x+y=w124:dbl)
                    n99 = Build Array(w124, w125) -> (w120:dbl[])
                    n100 = Build Array(w123, 0.0 ("element")) -> (w121:dbl[])
                    n101 = property on="tFit_array" class="Arr (strict)"("Value"=w121) -> ()  [unwired: 2 in, 2 out]
                    n102 = property on="PFit_array" class="Arr (strict)"("Value"=w120) -> ()  [unwired: 2 in, 2 out]
                  }
                }
              }
              frame #6 {
                n103 = property on="error" class="DigNum (strict)"() -> ("Value"=w137:dbl)  [unwired: 2 in, 2 out]
                n104 = property on="tPrev" class="DigNum (strict)"() -> ("Value"=w136:dbl)  [unwired: 2 in, 2 out]
                n105 = property on="tStart(s)" class="DigNum (strict)"() -> ("Value"=w135:dbl)  [unwired: 2 in, 2 out]
                n106 = Subtract(x=w135, y=w136) -> (x-y=w141:dbl)
                n107 = property on="dt(s)" class="DigNum (strict)"("Value"=w141) -> ()  [unwired: 2 in, 2 out]
                n108 = property on="integral" class="DigNum (strict)"() -> ("Value"=w139:dbl)  [unwired: 2 in, 2 out]
                n109 = Multiply(x=w137, y=w141) -> (x*y=w138:dbl)
                n110 = Add(x=w138, y=w139) -> (x+y=w140:dbl)
                n111 = property on="integral" class="DigNum (strict)"("Value"=w140) -> ()  [unwired: 2 in, 2 out]
              }
              frame #7 {
                n112 = property on="error" class="DigNum (strict)"() -> ("Value"=w154:dbl)  [unwired: 2 in, 2 out]
                n113 = property on="tune_Method" class="Ring (strict)"() -> ("Value"=w144:u16)  [unwired: 2 in, 2 out]
                n114 = property on="Kp" class="DigNum (strict)"() -> ("Value"=w143:dbl)  [unwired: 2 in, 2 out]
                n115 = property on="integral" class="DigNum (strict)"() -> ("Value"=w146:dbl)  [unwired: 2 in, 2 out]
                n116 = property on="derivative" class="DigNum (strict)"() -> ("Value"=w148:dbl)  [unwired: 2 in, 2 out]
                n117 = property on="Ki" class="DigNum (strict)"() -> ("Value"=w145:dbl)  [unwired: 2 in, 2 out]
                n118 = property on="Kd" class="DigNum (strict)"() -> ("Value"=w147:dbl)  [unwired: 2 in, 2 out]
                n119 = case shown="0, Default" w144 {
                  tunnel: w143 -> [w155 w158]
                  tunnel: [w155 w156] -> w142
                  frame 0, Default {
                  }
                  frame 1 {
                    n120 = Multiply(x=w158, y=-1.0) -> (x*y=w156:dbl)
                  }
                }
                n121 = Multiply(x=w147, y=w148) -> (x*y=w151:dbl)
                n122 = Multiply(x=w145, y=w146) -> (x*y=w150:dbl)
                n123 = Multiply(x=w142, y=w154) -> (x*y=w149:dbl)
                n124 = Add(x=w149, y=w150) -> (x+y=w152:dbl)
                n125 = Add(x=w152, y=w151) -> (x+y=w153:dbl)
                n126 = property on="dValue" class="DigNum (strict)"("Value"=w153) -> ()  [unwired: 2 in, 2 out]
              }
              frame #8 {
                n127 = property on="tuning" class="Bool (strict)"() -> ("Value"=w159:bool)  [unwired: 2 in, 2 out]
                n128 = case shown="True" w159 {
                  frame False {
                  }
                  frame True {
                    w172 = 90.0 ("y")
                    n129 = property on="current value" class="DigNum (strict)"() -> ("Value"=w178:dbl)  [unwired: 2 in, 2 out]
                    n130 = property on="dValue" class="DigNum (strict)"() -> ("Value"=w177:dbl)  [unwired: 2 in, 2 out]
                    n131 = Add(x=w178, y=w177) -> (x+y=w164:dbl)
                    "target value" <- w164
                    n132 = Less Than 0?(x=w164) -> (x < 0?=w176:bool)
                    n133 = Select(t=0.0, s=w176, f=w164) -> (s? t:f=w173:dbl)
                    n134 = Greater?(x=w173, y=w172) -> (0:w174:bool)
                    n135 = property on="tune_Method" class="Ring (strict)"() -> ("Value"=w163:u16)  [unwired: 2 in, 2 out]
                    n136 = property on="IO error" class="Clust (strict)"() -> ("Value"=w162:errorcluster)  [unwired: 2 in, 2 out]
                    n137 = Select(t=w172, s=w174, f=w173) -> (s? t:f=w161:dbl)
                    n138 = property on="current value" class="DigNum (strict)"("Value"=w161) -> ()  [unwired: 2 in, 2 out]
                    n139 = case shown="1" w163 {
                      tunnel: w162 -> [w182 w184]
                      tunnel: w161 -> [w181 w183]
                      tunnel: [w180 w185] -> w160
                      frame 0, Default {
                        n140 = property on="Tune Set Point (torr)" class="DigNum (strict)"("Value"=w181) -> ()  [unwired: 2 in, 2 out]
                        n141 = property on="Setpoint" class="Str"() -> ("Value"=w179:string)  [unwired: 2 in, 2 out]
                        n142 = call "writeSetPoint_00.vi"("error in"=w182, "P (Torr)"=w181, "Setpoint"=w179) -> ("error out"=w180:errorcluster)
                      }
                      frame 1 {
                        n143 = stacked-sequence {
                          tunnel: [_ _ _ w202] -> w185
                          tunnel: w184 -> [_ _ _ w201]
                          tunnel: w183 -> [_ w195 _ w199]
                          frame #0 {
                            n144 = property on="dAngle" class="DigNum (strict)"() -> ("Value"=w186:dbl)  [unwired: 2 in, 2 out]
                            n145 = property on="prev dAngle" class="DigNum (strict)"("Value"=w186) -> ()  [unwired: 2 in, 2 out]
                          }
                          frame #1 {
                            n146 = property on="Angle (deg)" class="DigNum (strict)"() -> ("Value"=w196:dbl)  [unwired: 2 in, 2 out]
                            n147 = Subtract(x=w195, y=w196) -> (x-y=w194:dbl)
                            n148 = property on="prev dAngle" class="DigNum (strict)"() -> ("Value"=w193:dbl)  [unwired: 2 in, 2 out]
                            n149 = property on="dAngle" class="DigNum (strict)"("Value"=w194) -> ()  [unwired: 2 in, 2 out]
                            n150 = Sign(1:w193) -> (0:w192:dbl)
                            n151 = Sign(1:w194) -> (0:w190:dbl)
                            n152 = Equal?(x=w190, y=w192) -> (x = y?=w191:bool)
                            n153 = Multiply(x=w190, y="|angle backlash|") -> (x*y=w188:dbl)
                            n154 = Negate(x=w188) -> (-x=w187:dbl)
                            n155 = property on="Move to ref angle first" class="Bool (strict)"("Value"=w191) -> ()  [unwired: 2 in, 2 out]
                            n156 = property on="angle backlash (deg)" class="DigNum (strict)"("Value"=w187) -> ()  [unwired: 2 in, 2 out]
                          }
                          frame #2 {
                          }
                          frame #3 {
                            n157 = property on="angle backlash (deg)" class="DigNum (strict)"() -> ("Value"=w197:dbl)  [unwired: 2 in, 2 out]
                            n158 = property on="Move to ref angle first" class="Bool (strict)"() -> ("Value"=w198:bool)  [unwired: 2 in, 2 out]
                            n159 = call "setAngleDir_07.vi"("Angle (deg)"=w199, "dAngle (deg)"=w197, "time to wait (s)"="time to wait (s)", "Move to ref angle first"=w198, "IO error in"=w201) -> ("IO error out"=w202:errorcluster)
                          }
                        }
                      }
                    }
                    n160 = property on="dt(s)" class="DigNum (strict)"() -> ("Value"=w170:dbl)  [unwired: 2 in, 2 out]
                    n161 = Subtract(x=w161, y=w164) -> (x-y=w171:dbl)
                    "windup error" <- w171
                    n162 = Multiply(x=w171, y=w170) -> (x*y=w169:dbl)
                    n163 = Multiply(x="Ks", y=w169) -> (x*y=w167:dbl)
                    n164 = property on="integral" class="DigNum (strict)"() -> ("Value"=w166:dbl)  [unwired: 2 in, 2 out]
                    n165 = Add(x=w167, y=w166) -> (x+y=w165:dbl)
                    n166 = property on="integral" class="DigNum (strict)"("Value"=w165) -> ()  [unwired: 2 in, 2 out]
                    n167 = property on="IO error" class="Clust (strict)"("Value"=w160) -> ()  [unwired: 2 in, 2 out]
                  }
                }
              }
              frame #9 {
                n168 = property on="Angle array" class="Arr (strict)"() -> ("Value"=w204:dbl[])  [unwired: 2 in, 2 out]
                n169 = property on="dt array" class="Arr (strict)"() -> ("Value"=w205:dbl[])  [unwired: 2 in, 2 out]
                n170 = property on="PFit_array" class="Arr (strict)"() -> ("Value"=w211:dbl[])  [unwired: 2 in, 2 out]
                n171 = property on="tFit_array" class="Arr (strict)"() -> ("Value"=w212:dbl[])  [unwired: 2 in, 2 out]
                n172 = property on="P array" class="Arr (strict)"() -> ("Value"=w213:dbl[])  [unwired: 2 in, 2 out]
                n173 = property on="Pset array" class="Arr (strict)"() -> ("Value"=w207:dbl[])  [unwired: 2 in, 2 out]
                n174 = Bundle("Value"=w205, "Value"=w204) -> (→"XY Graph 2":cluster{"Value":dbl[], "Value":dbl[]})  [unwired: 1 in]
                n175 = Bundle("Value"=w205, "Value"=w207) -> (w206:cluster{"Value":dbl[], "Value":dbl[]})  [unwired: 1 in]
                n176 = Bundle("Value"=w212, "Value"=w211) -> (w209:cluster{"Value":dbl[], "Value":dbl[]})  [unwired: 1 in]
                n177 = Bundle("Value"=w205, "Value"=w213) -> (w210:cluster{"Value":dbl[], "Value":dbl[]})  [unwired: 1 in]
                n178 = Build Array(w210, w209, w206) -> (→"XY Graph":cluster{"Value":dbl[], "Value":dbl[]}[])
              }
              frame #10 {
                n179 = property on="tStart(s)" class="DigNum (strict)"() -> ("Value"=w214:dbl)  [unwired: 2 in, 2 out]
                n180 = property on="tPrev" class="DigNum (strict)"("Value"=w214) -> ()  [unwired: 2 in, 2 out]
              }
            }
          }
          event "Hold": Value Change {
            n181 = event-data() -> ()  [unwired: 1 in, 5 out]
            n182 = property on="Hold" class="Bool (strict)"() -> ("Value"=w215:bool)  [unwired: 2 in, 2 out]
            n183 = case shown="False" w215 {
              frame False {
                n184 = property on="Local" class="Bool (strict)"() -> ("Value"=w216:bool)  [unwired: 2 in, 2 out]
                n185 = case shown="False" w216 {
                  frame False {
                    n186 = property on="IO error" class="Clust (strict)"() -> ("Value"=w220:errorcluster)  [unwired: 2 in, 2 out]
                    n187 = property on="Setpoint" class="Str"() -> ("Value"=w217:string)  [unwired: 2 in, 2 out]
                    n188 = call "readSetPoint00.vi"("error in"=w220, "Setpoint"=w217) -> ("error out"=w219:errorcluster, "P"=w218:dbl)
                    n189 = property on="Tune Set Point (torr)" class="DigNum (strict)"("Value"=w218) -> ()  [unwired: 2 in, 2 out]
                    n190 = property on="Set Point (torr)" class="DigNum (strict)"("Value"=w218) -> ()  [unwired: 2 in, 2 out]
                    n191 = property on="IO error" class="Clust (strict)"("Value"=w219) -> ()  [unwired: 2 in, 2 out]
                  }
                  frame True {
                  }
                }
              }
              frame True {
                n192 = property on="IO error" class="Clust (strict)"() -> ("Value"=w224:errorcluster)  [unwired: 2 in, 2 out]
                n193 = property on="Tune" class="Bool (strict)"("Value"=FALSE ("Tune")) -> ()  [unwired: 2 in, 2 out]
                n194 = property on="Local" class="Bool (strict)"("Value"=FALSE ("Local")) -> ()  [unwired: 2 in, 2 out]
                n195 = call "WriteAdaptorr03.vi"("error in (no error)"=w224, "string to write"="H") -> ("error out"=w223:errorcluster)
                n196 = property on="IO error" class="Clust (strict)"("Value"=w223) -> ()  [unwired: 2 in, 2 out]
              }
            }
          }
          event "Local": Value Change {
            n197 = event-data() -> ()  [unwired: 1 in, 5 out]
            n198 = property on="Local" class="Bool (strict)"() -> ("Value"=w226:bool)  [unwired: 2 in, 2 out]
            n199 = case shown="True" w226 {
              frame False {
                n200 = property on="IO error" class="Clust (strict)"() -> ("Value"=w229:errorcluster)  [unwired: 2 in, 2 out]
                n201 = call "WriteAdaptorr03.vi"("error in (no error)"=w229, "string to write"="H") -> ("error out"=w228:errorcluster)
                n202 = property on="Hold" class="Bool (strict)"("Value"=TRUE ("Hold")) -> ()  [unwired: 2 in, 2 out]
                n203 = property on="IO error" class="Clust (strict)"("Value"=w228) -> ()  [unwired: 2 in, 2 out]
              }
              frame True {
                n204 = property on="IO error" class="Clust (strict)"() -> ("Value"=w233:errorcluster)  [unwired: 2 in, 2 out]
                n205 = call "WriteAdaptorr03.vi"("error in (no error)"=w233, "string to write"="D5") -> ("error out"=w234:errorcluster)
                n206 = property on="Hold" class="Bool (strict)"("Value"=FALSE ("Hold")) -> ()  [unwired: 2 in, 2 out]
                n207 = property on="IO error" class="Clust (strict)"("Value"=w234) -> ()  [unwired: 2 in, 2 out]
              }
            }
          }
          event "Tune": Value Change {
            n208 = event-data() -> ()  [unwired: 1 in, 5 out]
            n209 = property on="Tune" class="Bool (strict)"() -> ("Value"=w235:bool)  [unwired: 2 in, 2 out]
            n210 = property on="tuning" class="Bool (strict)"("Value"=w235) -> ()  [unwired: 2 in, 2 out]
            n211 = case shown="True" w235 {
              frame False {
                n212 = property on="tune_Method" class="Ring (strict)"() -> ("Value"=w236:u16)  [unwired: 2 in, 2 out]
                n213 = case shown="1" w236 {
                  frame 0, Default {
                    n214 = property on="Set Point (torr)" class="DigNum (strict)"() -> ("Value"=w239:dbl)  [unwired: 2 in, 2 out]
                    n215 = property on="Setpoint" class="Str"() -> ("Value"=w240:string)  [unwired: 2 in, 2 out]
                    n216 = property on="IO error" class="Clust (strict)"() -> ("Value"=w238:errorcluster)  [unwired: 2 in, 2 out]
                    n217 = call "writeSetPoint_00.vi"("error in"=w238, "P (Torr)"=w239, "Setpoint"=w240) -> ("error out"=w237:errorcluster)
                    n218 = property on="IO error" class="Clust (strict)"("Value"=w237) -> ()  [unwired: 2 in, 2 out]
                  }
                  frame 1 {
                    n219 = flat-sequence {
                      frame #0 {
                        n220 = call "WriteAdaptorr03.vi"("string to write"="D5") -> ()  [unwired: 1 in, 1 out]
                      }
                      frame #1 {
                        n221 = property on="Setpoint" class="Str"() -> ("Value"=w243:string)  [unwired: 2 in, 2 out]
                        n222 = Concatenate Strings("Press ", w243, " on AdapTorr") -> (w242:string)
                        n223 = One Button Dialog(message=w242) -> ()  [unwired: 1 in, 1 out]
                      }
                    }
                  }
                }
              }
              frame True {
                n224 = property on="tune_Method" class="Ring (strict)"() -> ("Value"=w247:u16)  [unwired: 2 in, 2 out]
                n225 = case shown="0, Default" w247 {
                  frame 0, Default {
                    n226 = property on="IO error" class="Clust (strict)"() -> ("Value"=w250:errorcluster)  [unwired: 2 in, 2 out]
                    n227 = property on="Setpoint" class="Str"() -> ("Value"=w249:string)  [unwired: 2 in, 2 out]
                    n228 = call "readSetPoint00.vi"("error in"=w250, "Setpoint"=w249) -> ("error out"=w251:errorcluster, "P"=w248:dbl)
                    n229 = property on="Tune Set Point (torr)" class="DigNum (strict)"("Value"=w248) -> ()  [unwired: 2 in, 2 out]
                    n230 = property on="Set Point (torr)" class="DigNum (strict)"("Value"=w248) -> ()  [unwired: 2 in, 2 out]
                    n231 = property on="IO error" class="Clust (strict)"("Value"=w251) -> ()  [unwired: 2 in, 2 out]
                    n232 = property on="current value" class="DigNum (strict)"("Value"=w248) -> ()  [unwired: 2 in, 2 out]
                  }
                  frame 1 {
                    n233 = property on="Angle (deg)" class="DigNum (strict)"() -> ("Value"=w252:dbl)  [unwired: 2 in, 2 out]
                    n234 = property on="current value" class="DigNum (strict)"("Value"=w252) -> ()  [unwired: 2 in, 2 out]
                  }
                }
                n235 = property on="integral" class="DigNum (strict)"("Value"=0.0 ("integral")) -> ()  [unwired: 2 in, 2 out]
              }
            }
          }
          event "Set Point (torr)": Value Change {
            n236 = event-data() -> ()  [unwired: 1 in, 5 out]
            n237 = property on="Set Point (torr)" class="DigNum (strict)"() -> ("Value"=w255:dbl)  [unwired: 2 in, 2 out]
            n238 = property on="Setpoint" class="Str"() -> ("Value"=w256:string)  [unwired: 2 in, 2 out]
            n239 = property on="IO error" class="Clust (strict)"() -> ("Value"=w254:errorcluster)  [unwired: 2 in, 2 out]
            n240 = call "writeSetPoint_00.vi"("error in"=w254, "P (Torr)"=w255, "Setpoint"=w256) -> ("error out"=w253:errorcluster)
            n241 = property on="IO error" class="Clust (strict)"("Value"=w253) -> ()  [unwired: 2 in, 2 out]
          }
          event "Setpoint": Value Change {
            n242 = event-data() -> ()  [unwired: 1 in, 5 out]
            n243 = property on="Setpoint" class="Ring (strict)"() -> ("Value"=w261:u16)  [unwired: 2 in, 2 out]
            n244 = case shown="3" w261 {
              tunnel: ["A" "B" "C" "D"] -> w257
              frame 0, Default {
              }
              frame 1 {
              }
              frame 2 {
              }
              frame 3 {
              }
            }
            n245 = property on="Setpoint" class="Str"("Value"=w257) -> ()  [unwired: 2 in, 2 out]
            n246 = property on="IO error" class="Clust (strict)"() -> ("Value"=w258:errorcluster)  [unwired: 2 in, 2 out]
            n247 = call "readSetPoint00.vi"("error in"=w258, "Setpoint"=w257) -> ("error out"=w259:errorcluster, "P"=w260:dbl)
            n248 = property on="Set Point (torr)" class="DigNum (strict)"("Value"=w260) -> ()  [unwired: 2 in, 2 out]
            n249 = property on="Tune Set Point (torr)" class="DigNum (strict)"("Value"=w260) -> ()  [unwired: 2 in, 2 out]
            n250 = property on="IO error" class="Clust (strict)"("Value"=w259) -> ()  [unwired: 2 in, 2 out]
          }
          event "Method": Value Change {
            n251 = event-data() -> ()  [unwired: 1 in, 5 out]
            n252 = property on="Method" class="Ring (strict)"() -> ("Value"=w266:u16)  [unwired: 2 in, 2 out]
            n253 = case shown="1" w266 {
              frame 0, Default {
              }
              frame 1 {
                n254 = property on="tuning" class="Bool (strict)"() -> ("Value"=w267:bool)  [unwired: 2 in, 2 out]
                n255 = case shown="True" w267 {
                  frame False {
                  }
                  frame True {
                    n256 = flat-sequence {
                      frame #0 {
                        n257 = call "WriteAdaptorr03.vi"("string to write"="D5") -> ()  [unwired: 1 in, 1 out]
                      }
                      frame #1 {
                        n258 = property on="Setpoint" class="Str"() -> ("Value"=w270:string)  [unwired: 2 in, 2 out]
                        n259 = Concatenate Strings("Press ", w270, " on AdapTorr") -> (w269:string)
                        n260 = One Button Dialog(message=w269) -> ()  [unwired: 1 in, 1 out]
                      }
                    }
                  }
                }
              }
            }
            n261 = property on="tune_Method" class="Ring (strict)"("Value"=w266) -> ()  [unwired: 2 in, 2 out]
          }
        }
      }
    }
    frame #2 {
      n262 = property on="tuning" class="Bool (strict)"() -> ("Value"=w273:bool)  [unwired: 2 in, 2 out]
      n263 = case shown="True" w273 {
        frame False {
        }
        frame True {
          n264 = property on="tune_Method" class="Ring (strict)"() -> ("Value"=w274:u16)  [unwired: 2 in, 2 out]
          n265 = case shown="1" w274 {
            frame 0, Default {
            }
            frame 1 {
              n266 = flat-sequence {
                frame #0 {
                  n267 = property on="IO error" class="Clust (strict)"() -> ("Value"=w276:errorcluster)  [unwired: 2 in, 2 out]
                  n268 = call "setLocal_And_Hold_00.vi"("error in (no error)"=w276) -> ("error out"=w275:errorcluster)
                  n269 = property on="IO error" class="Clust (strict)"("Value"=w275) -> ()  [unwired: 2 in, 2 out]
                }
                frame #1 {
                  n270 = property on="Setpoint" class="Str"() -> ("Value"=w278:string)  [unwired: 2 in, 2 out]
                  n271 = Concatenate Strings("Press ", w278, " on AdapTorr") -> (w277:string)
                  n272 = One Button Dialog(message=w277) -> ()  [unwired: 1 in, 1 out]
                }
              }
            }
          }
        }
      }
    }
  }
